vi "GATES.vi"() -> ()   [LabVIEW 2018]
panel:
  out "OUTPUT":dbl
  in  "Numeric 2":dbl
  in  "Numeric":dbl
  in  "Tab Control":T1(tab)
  in  "AND GATE":string[][](table)=[["X", "Y", "OUTPUT"], ["0", "0", ""], ["0", "1", ""], ["1", "0", ""], ["1", "1", ""]]
  out "AND":bool
  in  "OR GATE":string[][](table)
  out "OR":bool
  in  "NOT GATE":string[][](table)
  out "NOT":bool
  in  "NAND GATE":string[][](table)
  out "NAND":bool
  in  "NOR GATE":string[][](table)
  out "NOR":bool
  in  "XOR GATE":string[][](table)
  out "XOR":bool
  in  "X NOR GATE":string[][](table)
  out "XNOR":bool
  in  "IMPLIES":string[][](table)
  out "IMPLIES 2":bool
  in  "B":bool
  in  "A":bool
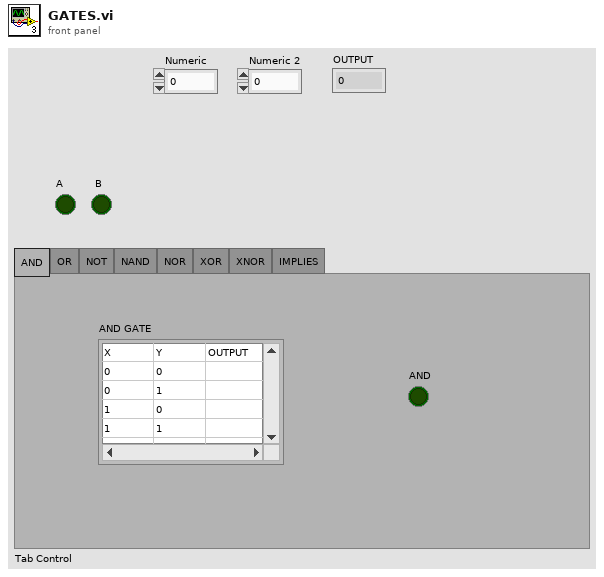
[diagram p1: front panel]
types:
  T1 = enum32{"AND", "OR", "NOT", "NAND", "NOR", "XOR", "XNOR", "IMPLIES"}
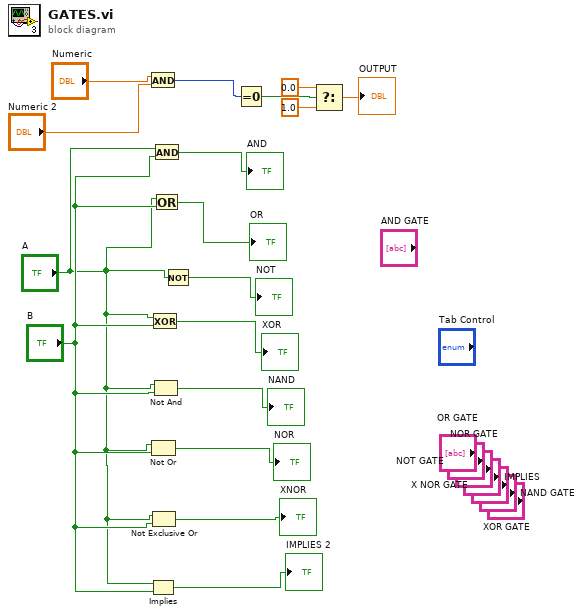
[diagram p0: block diagram]
diagram:
  n1 = And(x="Numeric", y="Numeric 2") -> (x .and. y?=w5:i32)
  n2 = Not Or(1:"B", 2:"A") -> (0:→"NOR":bool)
  n3 = Implies(1:"B", 2:"A") -> (0:→"IMPLIES 2":bool)
  n4 = Not Exclusive Or(1:"B", 2:"A") -> (0:→"XNOR":bool)
  n5 = Exclusive Or(1:"B", 2:"A") -> (0:→"XOR":bool)
  n6 = Not And(1:"B", 2:"A") -> (0:→"NAND":bool)
  n7 = And(x="A", y="B") -> (x .and. y?=→"AND":bool)
  n8 = Or(x="A", y="B") -> (x .or. y?=→"OR":bool)
  n9 = Not(x="A") -> (.not. x?=→"NOT":bool)
  n10 = Equal To 0?(x=w5) -> (x = 0?=w4:bool)
  n11 = Select(t=0.0, s=w4, f=1.0) -> (s? t:f=→"OUTPUT":dbl)
